vi "Database Driver LV.vi"(4 "Create Table":T4={"table"="", "column information"=[], "primary key (-1)"=-1, "use file? (F)"=FALSE}, 5 "Insert Data":T1, 6 "Options":T6=enum."Select Data", 7 "SQLTableData":T5, 8 "error in":errorcluster, 9 "SQL query":string, 10 "Select":enum16{"SelectWithQuery", "SelectWithColumn"}(ring), 11 "table":string) -> (0 "error out":errorcluster, 1 "tables":string[](array[string]), 2 "Database out":refnum<class "Database.lvclass">, 3 "data":string[][](array[string]))   [LabVIEW 2023, in "HardwareAbstractionLayer_LVOOP.lvlib" / "Database.lvclass"]
doc: "This VI used to Database action engine.\n\n// Defeault Case Select Query"
uses:
  Database.lvclass
  Control/DB Options.ctl
  <vilib>/addons/database/Auxilliary.llb/DB Tools Column Info.ctl
  <vilib>/addons/database/Auxilliary.llb/DB Tools DataTypes.ctl
  Control/DB Selection.ctl
  MYSQL Database_class/MYSQL Database.lvclass
  SQLite Database_class/SQLite Database.lvclass
  Database.lvclass/Database.ctl
  <vilib>/addons/database/NI_Database_API.lvlib
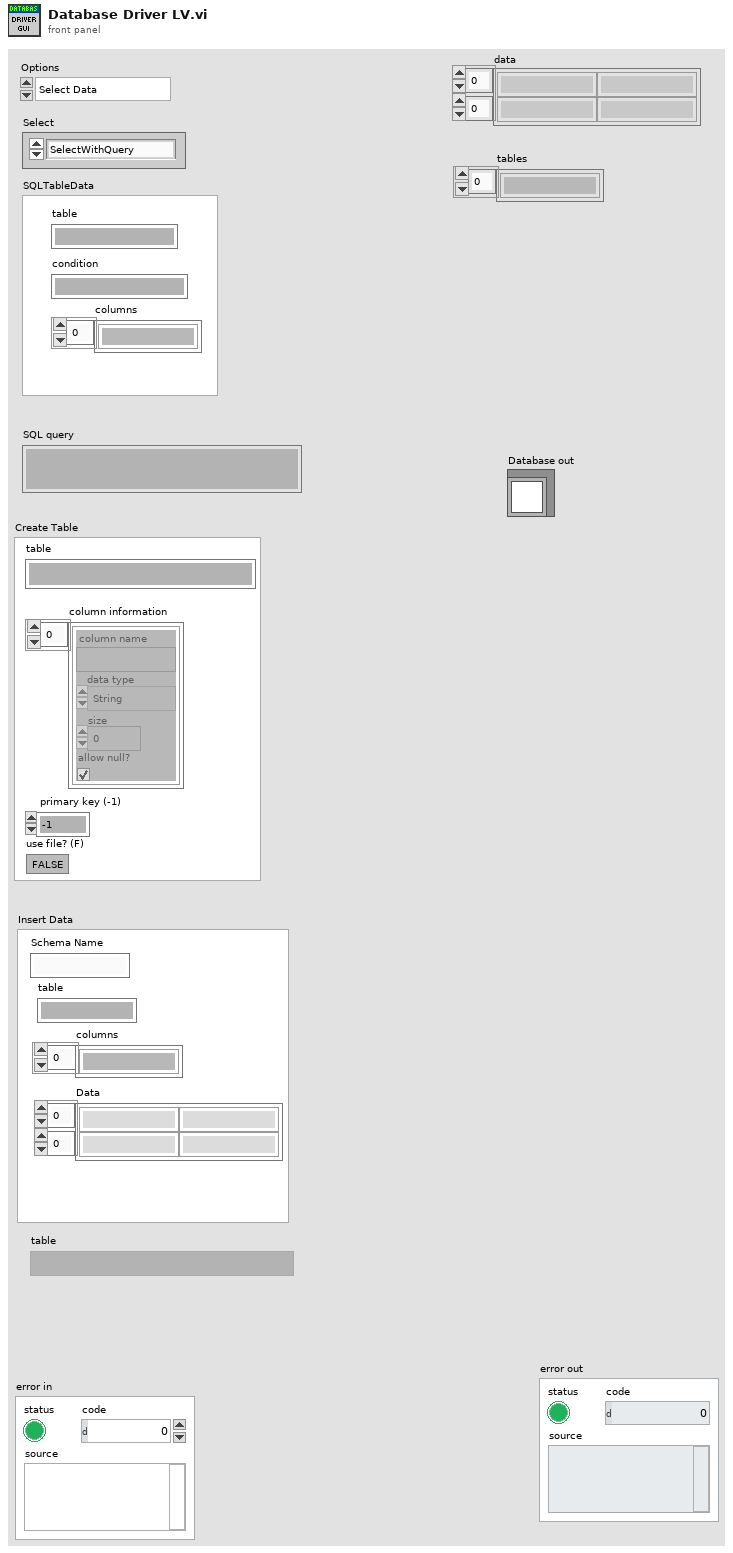
[diagram p1: front panel]
types:
  T1 = cluster{"table":string, "columns":string[], "Data":string[][], "Schema Name":string}
  T2 = typedef "NI_Database_API.lvlib/DB Tools Column Info.ctl" = cluster{"column name":string, "data type":T3, "size":i32, "allow null?":bool}
  T3 = typedef "NI_Database_API.lvlib/DB Tools DataTypes.ctl" = enum16{"String", "Long (I32)", "Single (SGL)", "Double (DBL)", "Date/Time", "Binary"}
  T4 = cluster{"table":string, "column information":T2[], "primary key (-1)":i32, "use file? (F)":bool}
  T5 = cluster{"table":string, "condition":string, "columns":string[]}
  T6 = typedef "HardwareAbstractionLayer_LVOOP.lvlib/Database.lvclass/DB Options.ctl" = enum16{"Init", "Select Data", "Insert Data", "Update Data", "Delete Data", "Execute Query", "Create Schema", "Create Table", "List Tables", "List Columns", "Close"}
  T7 = cluster{"DataSource Name":string, "userID":string, "password":string}
  T8 = enum16{"open", "replace", "create", "open or create", "replace or create", "replace or create with confirmation"}
  T9 = typedef "HardwareAbstractionLayer_LVOOP.lvlib/Database.lvclass/DB Selection.ctl" = string
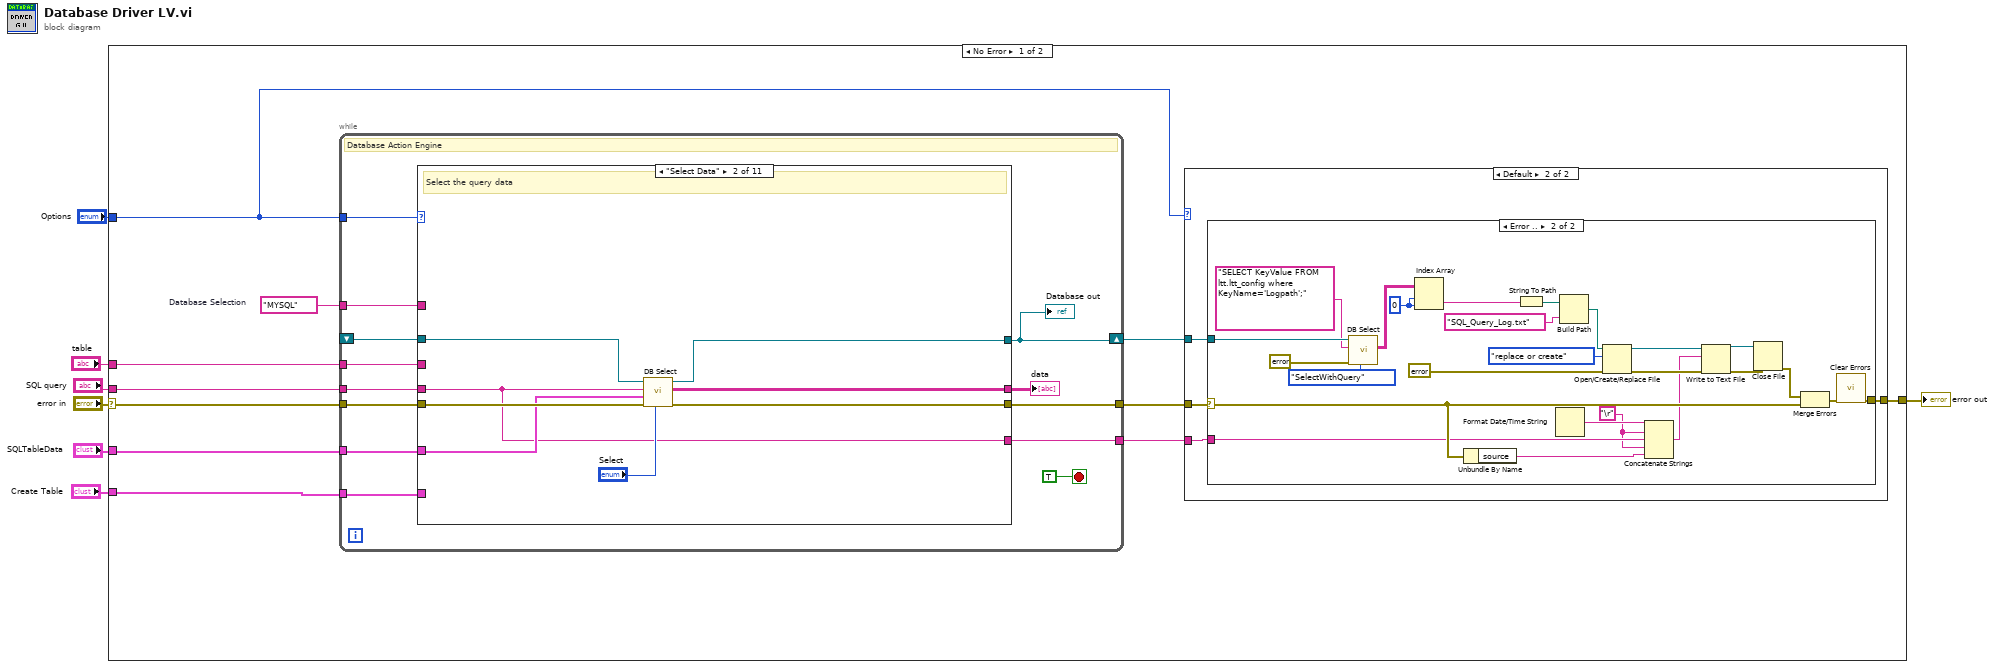
[diagram p0: block diagram]
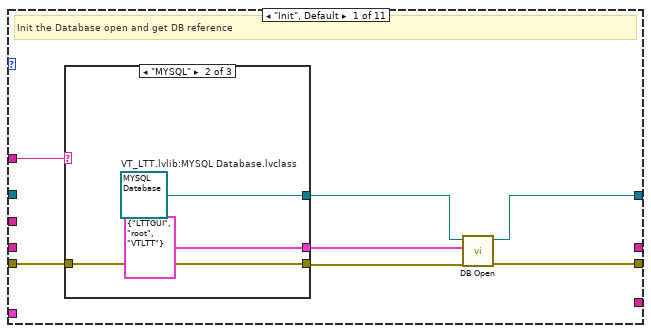
[diagram p2: hidden frame]
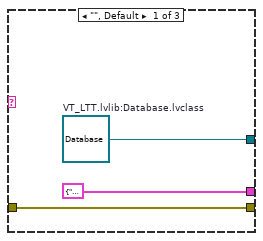
[diagram p3: hidden frame]
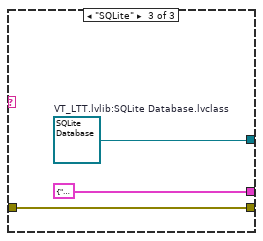
[diagram p4: hidden frame]
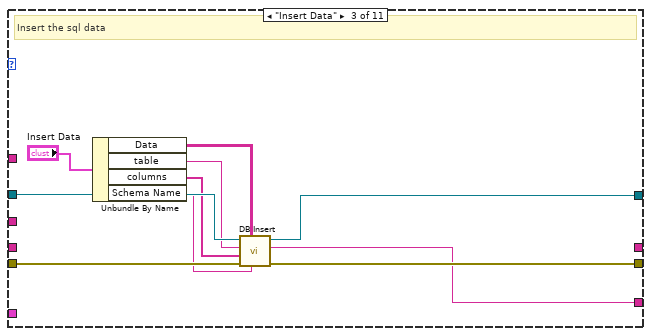
[diagram p5: hidden frame]
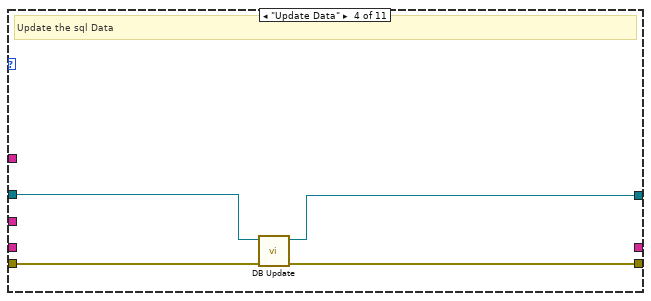
[diagram p6: hidden frame]
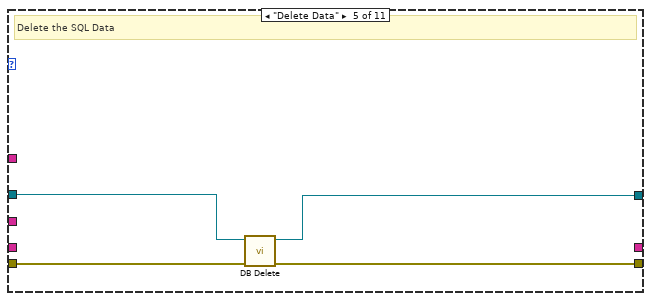
[diagram p7: hidden frame]
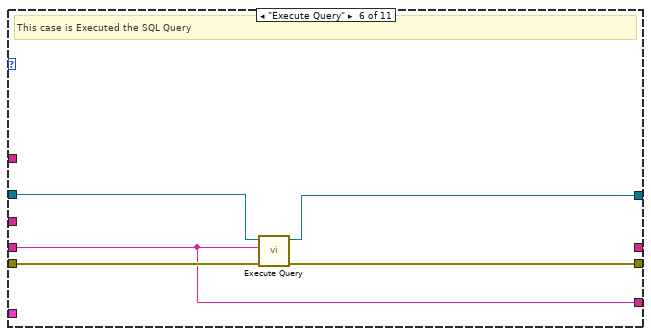
[diagram p8: hidden frame]
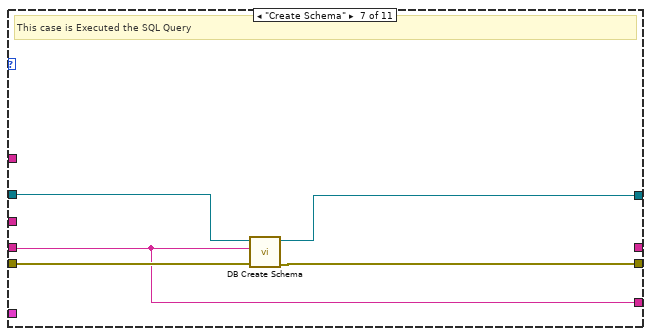
[diagram p9: hidden frame]
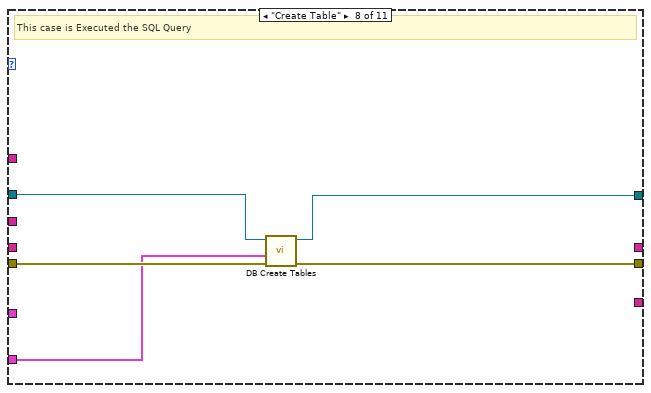
[diagram p10: hidden frame]
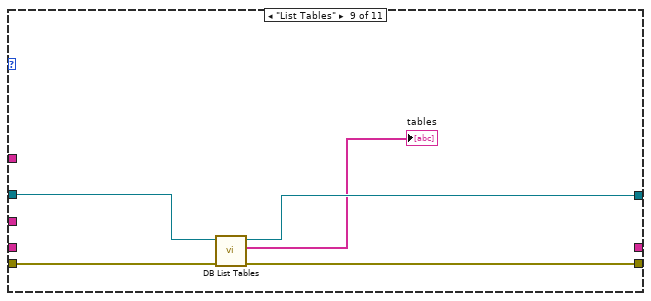
[diagram p11: hidden frame]
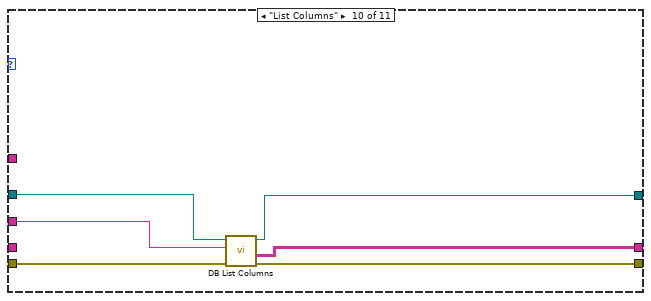
[diagram p12: hidden frame]
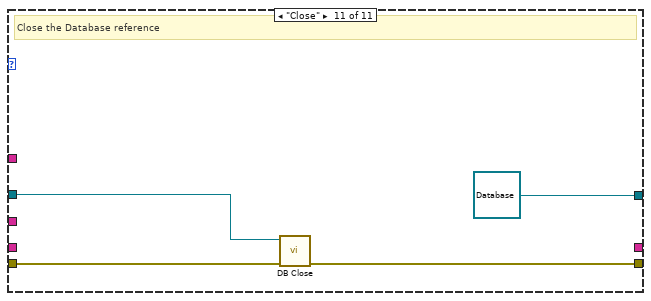
[diagram p13: hidden frame]
diagram:
  n1 = case shown="No Error" "error in" {
    selector: "error in" -> [w17 w135]
    tunnel: "SQL query" -> [w16 _]
    tunnel: "SQLTableData" -> [w15 _]
    tunnel: "Create Table" -> [w14 _]
    tunnel: "table" -> [w13 _]
    tunnel: [w10 w135] -> w2
    tunnel: "Options" -> [w9 _]
    frame No Error {
      w18 = T9 "MYSQL"  # Database Selection
      n2 = while {
        tunnel: w9 -> [w30]
        tunnel: w18 -> [w29]
        shift-right: [w21] -> w8
        shift-left: _ -> [w26]
        tunnel: w16 -> [w25]
        tunnel: w15 -> [w24]
        tunnel: w14 -> [w22]
        tunnel: w13 -> [w20]
        tunnel: [w19] -> w11
        tunnel: w17 -> [w28]
        tunnel: [w27] -> w12
        stop <- TRUE stop-if-true
        # "Database Action Engine"
        n3 = case shown="\"Select Data\"" w30 {
          tunnel: w29 -> [w38 _ _ _ _ _ _ _ _ _ _]
          tunnel: w28 -> [w37 w55 w64 w69 w73 w78 w82 w86 w92 w98 w103]
          tunnel: [w32 w54 w63 w68 w72 w77 w81 w85 w91 w96 w102] -> w27
          tunnel: [w33 w52 w62 w66 w70 w75 w80 w87 w90 w97 refnum<class "Database.lvclass"> refnum ("Database out")] -> w21
          tunnel: w26 -> [_ w53 w65 w67 w71 w76 w83 w88 w93 w99 w101]
          tunnel: w25 -> [_ w48 _ _ _ w74 w79 _ _ _ _]
          tunnel: w24 -> [_ w50 _ _ _ _ _ _ _ _ _]
          tunnel: [_ w49 _ _ _ _ _ _ _ w94 _] -> w23
          tunnel: w22 -> [_ _ _ _ _ _ _ w84 _ _ _]
          tunnel: w20 -> [_ _ _ _ _ _ _ _ _ w95 _]
          tunnel: [_ w48 w56 _ _ w74 w79 _ _ _ _] -> w19
          frame "Init", Default {
            # "Init the Database open and get DB reference"
            n4 = case shown="\"MYSQL\"" w38 {
              tunnel: w37 -> [w41 w44 w47]
              tunnel: [w41 w44 w47] -> w36
              tunnel: [w40 w43 w46] -> w35
              tunnel: [T7 {"DataSource Name"="", "userID"="", "password"=""} ("DB") T7 {"DataSource Name"="LTTGUI", "userID"="root", "password"="VTLTT"} ("DB") T7 {"DataSource Name"="", "userID"="", "password"=""} ("DB")] -> w34
              frame "", Default {
                w40 = refnum<class "Database.lvclass"> refnum  # VT_LTT.lvlib:Database.lvclass
              }
              frame "MYSQL" {
                w43 = refnum<class "MYSQL Database.lvclass"> refnum  # VT_LTT.lvlib:MYSQL Database.lvclass
              }
              frame "SQLite" {
                w46 = refnum<class "SQLite Database.lvclass"> refnum  # VT_LTT.lvlib:SQLite Database.lvclass
              }
            }
            n5 = call-dynamic "DB Open.vi"("error in"=w36, "DB"=w34, "Database in"=w35) -> ("error out"=w32:errorcluster, "Database out"=w33:refnum<class "Database.lvclass">)  [unwired: 7 in]
          }
          frame "Select Data" {
            # "Select the query data"
            n6 = call-dynamic "DB Select.vi"("Select"="Select", "error in (no error)"=w55, "SQLTableData"=w50, "SQL query"=w48, "Database in"=w53) -> ("error out"=w54:errorcluster, "data"=w49:string[][], "Database out"=w52:refnum<class "Database.lvclass">)  [unwired: 4 in]
          }
          frame "Insert Data" {
            # "Insert the sql data"
            n7 = Unbundle By Name("Insert Data") -> ("Data"=w58:string[][], "table"=w60:string, "columns"=w59:string[], "Schema Name"=w57:string)
            n8 = call-dynamic "DB Insert.vi"("Schema Name"=w57, "Data"=w58, "error in (no error)"=w64, "columns"=w59, "table"=w60, "Database in"=w65) -> ("error out"=w63:errorcluster, "SQL"=w56:string, "Database out"=w62:refnum<class "Database.lvclass">)  [unwired: 3 in]
          }
          frame "Update Data" {
            # "Update the sql Data"
            n9 = call-dynamic "DB Update.vi"("error in (no error)"=w69, "Database in"=w67) -> ("error out"=w68:errorcluster, "Database out"=w66:refnum<class "Database.lvclass">)  [unwired: 8 in]
          }
          frame "Delete Data" {
            # "Delete the SQL Data"
            n10 = call-dynamic "DB Delete.vi"("error in (no error)"=w73, "Database in"=w71) -> ("error out"=w72:errorcluster, "Database out"=w70:refnum<class "Database.lvclass">)  [unwired: 8 in]
          }
          frame "Execute Query" {
            # "This case is Executed the SQL Query"
            n11 = call-dynamic "Execute Query.vi"("error in (no error)"=w78, "SQL query"=w74, "Database in"=w76) -> ("error out"=w77:errorcluster, "Database out"=w75:refnum<class "Database.lvclass">)  [unwired: 7 in]
          }
          frame "Create Schema" {
            # "This case is Executed the SQL Query"
            n12 = call-dynamic "DB Create Schema.vi"("error in (no error)"=w82, "SQL query"=w79, "Database in"=w83) -> ("error out"=w81:errorcluster, "Database out"=w80:refnum<class "Database.lvclass">)  [unwired: 7 in]
          }
          frame "Create Table" {
            # "This case is Executed the SQL Query"
            n13 = call-dynamic "DB Create Tables.vi"("error in (no error)"=w86, "Create Table"=w84, "Database in"=w88) -> ("error out"=w85:errorcluster, "Database out"=w87:refnum<class "Database.lvclass">)  [unwired: 7 in]
          }
          frame "List Tables" {
            n14 = call-dynamic "DB List Tables.vi"("error in (no error)"=w92, "Database in"=w93) -> ("error out"=w91:errorcluster, "tables"=→"tables":string[], "Database out"=w90:refnum<class "Database.lvclass">)  [unwired: 7 in]
          }
          frame "List Columns" {
            n15 = call-dynamic "DB List Columns.vi"("error in (no error)"=w98, "table"=w95, "Database in"=w99) -> ("error out"=w96:errorcluster, "tableDetails"=w94:string[][], "Database out"=w97:refnum<class "Database.lvclass">)  [unwired: 5 in, 1 out]
          }
          frame "Close" {
            # "Close the Database reference"
            n16 = call-dynamic "DB Close.vi"("error in"=w103, "Database in"=w101) -> ("error out"=w102:errorcluster)  [unwired: 8 in, 1 out]
          }
        }
        "data" <- w23
        "Database out" <- w21
      }
      n17 = case shown="Default" w9 {
        tunnel: w12 -> [w104 w108]
        tunnel: w11 -> [_ w107]
        tunnel: [w104 w106] -> w10
        tunnel: w8 -> [_ w105]
        frame "Init", "Close" {
        }
        frame Default {
          n18 = case shown="Error .." w108 {
            selector: w108 -> [w109 w116]
            tunnel: w107 -> [_ w113]
            tunnel: [w109 w110] -> w106
            tunnel: w105 -> [_ w125]
            frame No Error {
            }
            frame Error {
              w112 = "\r"
              w121 = 0 ("disabled index (col)")
              n19 = call-dynamic "DB Select.vi"("Select"=enum16{"SelectWithQuery", "SelectWithColumn"}."SelectWithQuery", "error in (no error)"=errorcluster {"status"=FALSE, "code"=0, "source"=""}, "SQL query"="SELECT KeyValue FROM ltt.ltt_config where KeyName='Logpath';", "Database in"=w125) -> ("data"=w122:string[][])  [unwired: 5 in, 2 out]
              n20 = Index Array(array=w122, index (row)=w121, index (col)=w121) -> (element=w120:string)
              n21 = Unbundle By Name(w116) -> ("source"=w111:string)
              n22 = String To Path(string=w120) -> (path=w119:path)
              n23 = Format Date/Time String() -> (date/time string=w115:string)  [unwired: 3 in]
              n24 = Build Path(base path=w119, name or relative path="SQL_Query_Log.txt") -> (appended path=w128:path)
              n25 = Open/Create/Replace File(file path (use dialog)=w128, error in=errorcluster {"status"=FALSE, "code"=0, "source"=""}, operation (0:open)=T8."replace or create") -> (refnum out=w132:refnum<file>, error out=w131:errorcluster)  [unwired: 3 in, 1 out]
              n26 = Concatenate Strings(w115, w112, w113, w112, w111) -> (w114:string)
              n27 = Write to Text File(file (use dialog)=w132, text=w114, error in=w131) -> (refnum out=w134:refnum<file>, error out=w133:errorcluster)  [unwired: 1 in, 1 out]
              n28 = Close File(refnum=w134, error in=w133) -> (error out=w127:errorcluster)  [unwired: 1 out]
              n29 = Merge Errors(w127, w116) -> (w126:errorcluster)
              n30 = call <vilib>:"Clear Errors.vi"("error in (no error)"=w126) -> ("error out"=w110:errorcluster)  [unwired: 5 in, 1 out]
            }
          }
        }
      }
    }
    frame Error {
    }
  }
  "error out" <- w2
